vi "2 inputs loop trial.vi"() -> ()   [LabVIEW 2015]
doc: "This example VI shows how to convert string data elements to numeric elements so it can be graphed and displayed on an XY Graph."
uses:
  <instrlib>/Keithley 27XX/Public/Data/Read Multiple Direct.vi
  <instrlib>/Keithley 27XX/Keithley 27XX.lvlib
panel:
  out "Array":dbl[](array[numeric])
  out "Waveform Chart 4":dbl(graph)
  out "Waveform Chart 3":dbl(graph)
  out "Waveform Chart 2":dbl(graph)
  out "Waveform Chart":dbl(graph)
  out "element 2":dbl
  out "element":dbl
  in  "Number of channels":i32=1
  in  "Function (6: Temp)":u16(ring)=6 items=["DC Voltage", "AC Voltage", "DC Current", "AC Current", "Resistance", "Four-Wire Resistance", "Temperature (C)", "Frequency", "Period", "Continuity"]
  in  "Sample Count (10)":i32=10
  in  "Channel List (101)":string="101"
  in  "Serial Configuration":T1={"Baud Rate (9600)"=9600, "Flow Control (1: XON/XOFF)"=1, "Termination Char (0:CR)"=0} {"Termination Char (0:CR)" items=["CR", "LF", "CRLF (Do not use)", "LFCR (Do not use)"]; "Flow Control (1: XON/XOFF)" items=["None", "XON/XOFF", "RTS/CTS (2701 Only)", "XON/XOFF & RTS/CTS (2701 Only)"]; "Baud Rate (9600)" items=["300"=300, "600"=600, "1200"=1200, "2400"=2400, "4800"=4800, "9600"=9600, "19.2k"=19200, "38.4k (2701 Only)"=38400, "57.6k (2701 Only)"=57600, "115.2k (2701 Only)"=115200]}
  in  "VISA resource name":refnum<visa-resource-name>="GPIB0::19::INSTR"
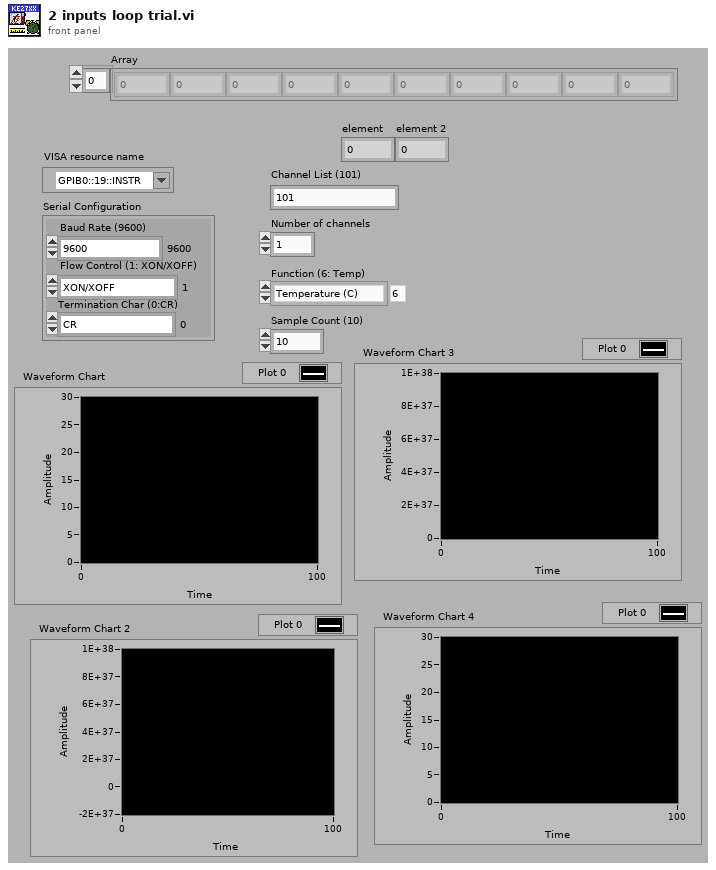
[diagram p1: front panel]
types:
  T1 = cluster{"Baud Rate (9600)":u32, "Flow Control (1: XON/XOFF)":u16, "Termination Char (0:CR)":u16}
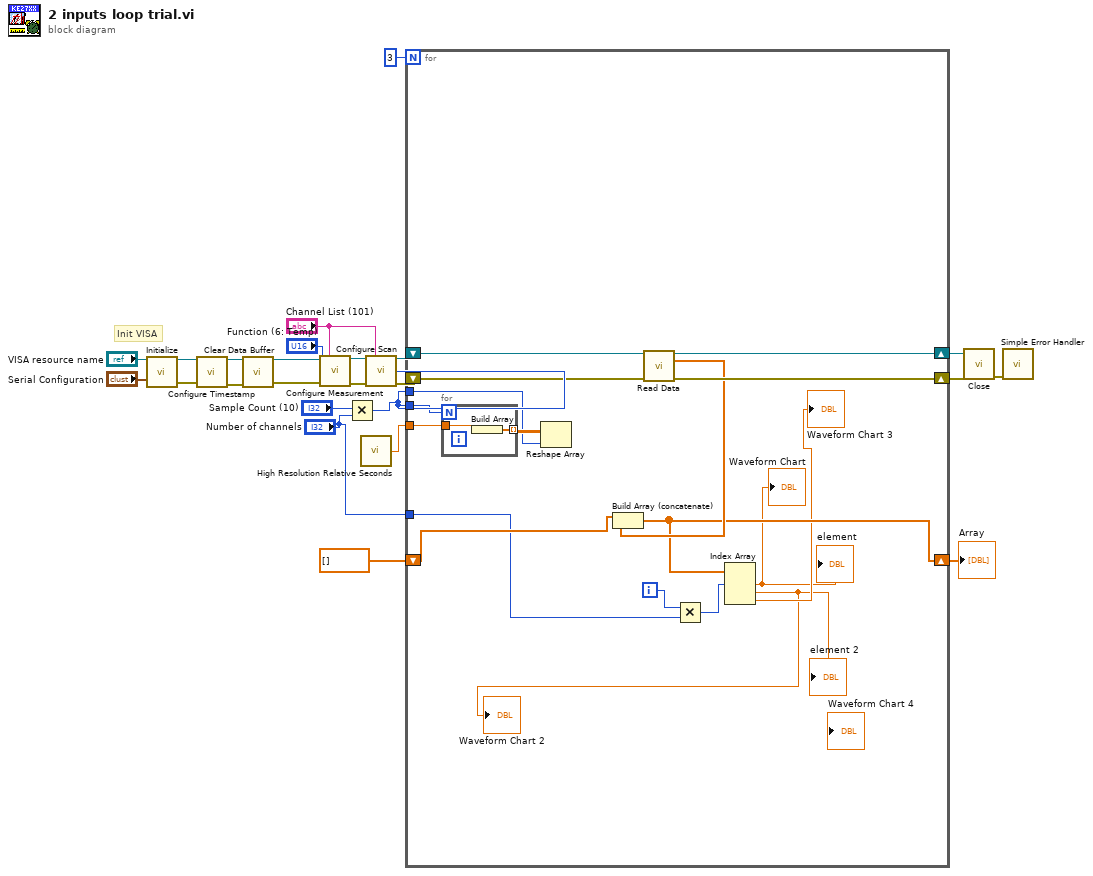
[diagram p0: block diagram]
diagram:
  # "Init VISA"
  n1 = call <instrlib>:"Initialize.vi"("VISA resource name"="VISA resource name", "Serial Configuration"="Serial Configuration") -> ("VISA resource name out"=w21:refnum<visa-resource-name>, "error out"=w20:errorcluster)  [unwired: 12 in]
  n2 = call <instrlib>:"Configure Timestamp.vi"("VISA resource name"=w21, "error in (no error)"=w20) -> ("VISA resource name out"=w16:refnum<visa-resource-name>, "error out"=w15:errorcluster)  [unwired: 12 in]
  n3 = call <instrlib>:"Clear Data Buffer.vi"("VISA resource name"=w16, "error in (no error)"=w15) -> ("VISA resource name out"=w14:refnum<visa-resource-name>, "error out"=w17:errorcluster)  [unwired: 12 in]
  n4 = call <instrlib>:"Configure Measurement.vi"("VISA resource name"=w14, "Scan List (Empty)"="Channel List (101)", "Function (0: DC Voltage)"="Function (6: Temp)", "error in (no error)"=w17) -> ("VISA resource name out"=w13:refnum<visa-resource-name>, "error out"=w11:errorcluster)  [unwired: 10 in]
  n5 = Multiply(x="Sample Count (10)", y="Number of channels") -> (x*y=w5:i32)
  n6 = call <vilib>:"High Resolution Relative Seconds.vi"() -> ("relative seconds"=w7:dbl)
  n7 = call <instrlib>:"Configure Scan.vi"("VISA resource name"=w13, "Channel List (101:110)"="Channel List (101)", "Sample Count (100)"=w5, "error in (no error)"=w11) -> ("VISA resource name out"=w9:refnum<visa-resource-name>, "error out"=w8:errorcluster)  [unwired: 10 in]
  n8 = for {
    N: 3 -> [_]
    shift-right: [w40] -> w18
    shift-left: w9 -> [w39]
    shift-right: [w41] -> w19
    shift-left: w8 -> [w38]
    tunnel: w5 -> [w37]
    tunnel: w7 -> [w36]
    tunnel: w5 -> [w34]
    tunnel: "Number of channels" -> [w29]
    shift-right: [w31] -> w1
    shift-left: dbl[] [] -> [w32]
    i -> [w30]
    n9 = for {
      N: w37 -> [_]
      tunnel: w36 -> [w43]
      tunnel: [w42] -> w35 mode=indexing
      n10 = Build Array(w43) -> (w42:dbl[])
    }
    n11 = Reshape Array(w35, w34) -> ()  [unwired: 1 out]
    n12 = call-poly <instrlib>:"Read Data.vi"("VISA resource name"=w39, "error in (no error)"=w38) -> ("VISA resource name out"=w40:refnum<visa-resource-name>, "Measurement Data"=w33:dbl[], "error out"=w41:errorcluster)  [unwired: 8 in, 3 out]
    n13 = Build Array (concatenate)(w32, w33) -> (w31:dbl[])
    n14 = Multiply(x=w30, y=w29) -> (x*y=w28:i32)
    n15 = Index Array(array=w31, index #1=w28) -> (element #1=→"element" →"Waveform Chart":dbl, element #2=→"element 2" →"Waveform Chart 2":dbl, element #3=→"Waveform Chart 3":dbl)  [unwired: 2 in]
  }
  "Array" <- w1
  n16 = call <instrlib>:"Close.vi"("VISA resource name"=w18, "error in (no error)"=w19) -> ("error out"=w22:errorcluster)  [unwired: 13 in]
  n17 = call <vilib>:"Simple Error Handler.vi"("error in (no error)"=w22) -> ()  [unwired: 4 in, 5 out]
